vi "Newport ITX-D3N.vi"(5 "Disable Filter?":bool, 7 "Device Number (Display In Header)":string, 8 "error in (no error)":errorcluster, 10 "Remote Port":u16=2000, 11 "Machine":string="192.168.1.200") -> (0 "error out":errorcluster, 1 "iTHX/iBTHX Output":T1, 2 "Newport ITX Data":string[][](array[string]), 3 "Temp/Humidity":dbl[](array[numeric]))   [LabVIEW 2019]
doc: "Demonstrates how to display an interactive send and receive message dialog for communication between TCP connections. It establishes a connection on the machine listed and the port specified. It then waits for you to input data into the Input Line string control and hit enter. Once you hit enter, the string you typed is sent to the port and passed to the TCP Communicator - Passive.vi where it is displayed on a string indicator.\n\nThe key difference between the Active and Passive VIs is that the Active VI establishes a connection, while the Passive VI waits for a connection to be established.\n\n<B>Note:</B> Requires the TCP Communicator - Passive.vi."
uses:
  Type Definitions/iBTHX Data Values.ctl
panel:
  out "error out 2":errorcluster
  # "Instructions:\n1. Open the TCP\n    Communicator - Passive.vi\n    and run it first.\n2. Run TCP Communicator - \n    Active.vi second.\n3.Type into the Input Line\n    String Control and then\n    hit Enter.\n4. Type into the Input Line\n    of the other VI and then\n    hit Enter.\n5. Press Stop to end session."
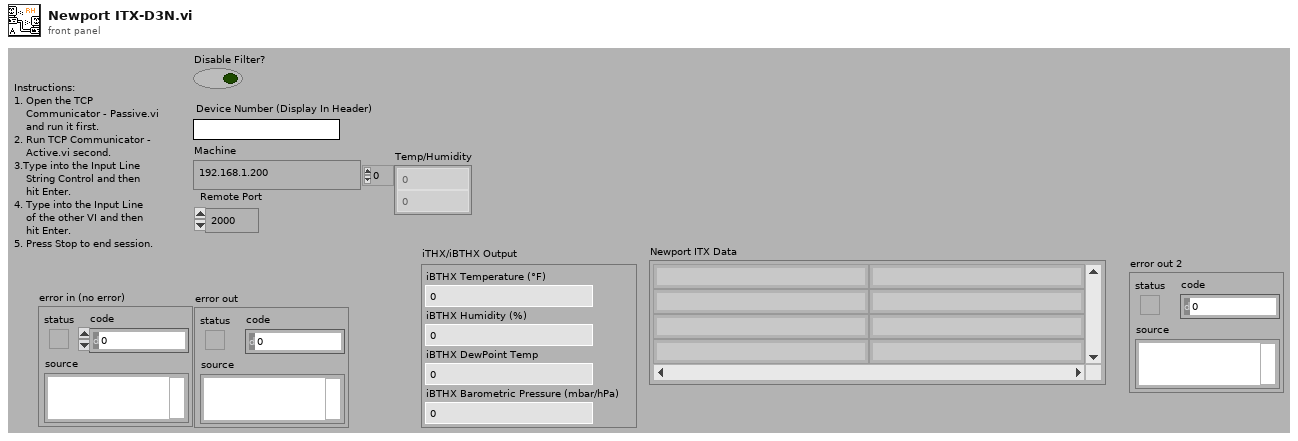
[diagram p1: front panel]
types:
  T1 = typedef "iBTHX Data Values.ctl" = cluster{"iBTHX Barometric Pressure (mbar/hPa)":dbl, "iBTHX Humidity (%)":dbl, "iBTHX Temperature (°F)":dbl, "iBTHX DewPoint Temp":dbl}
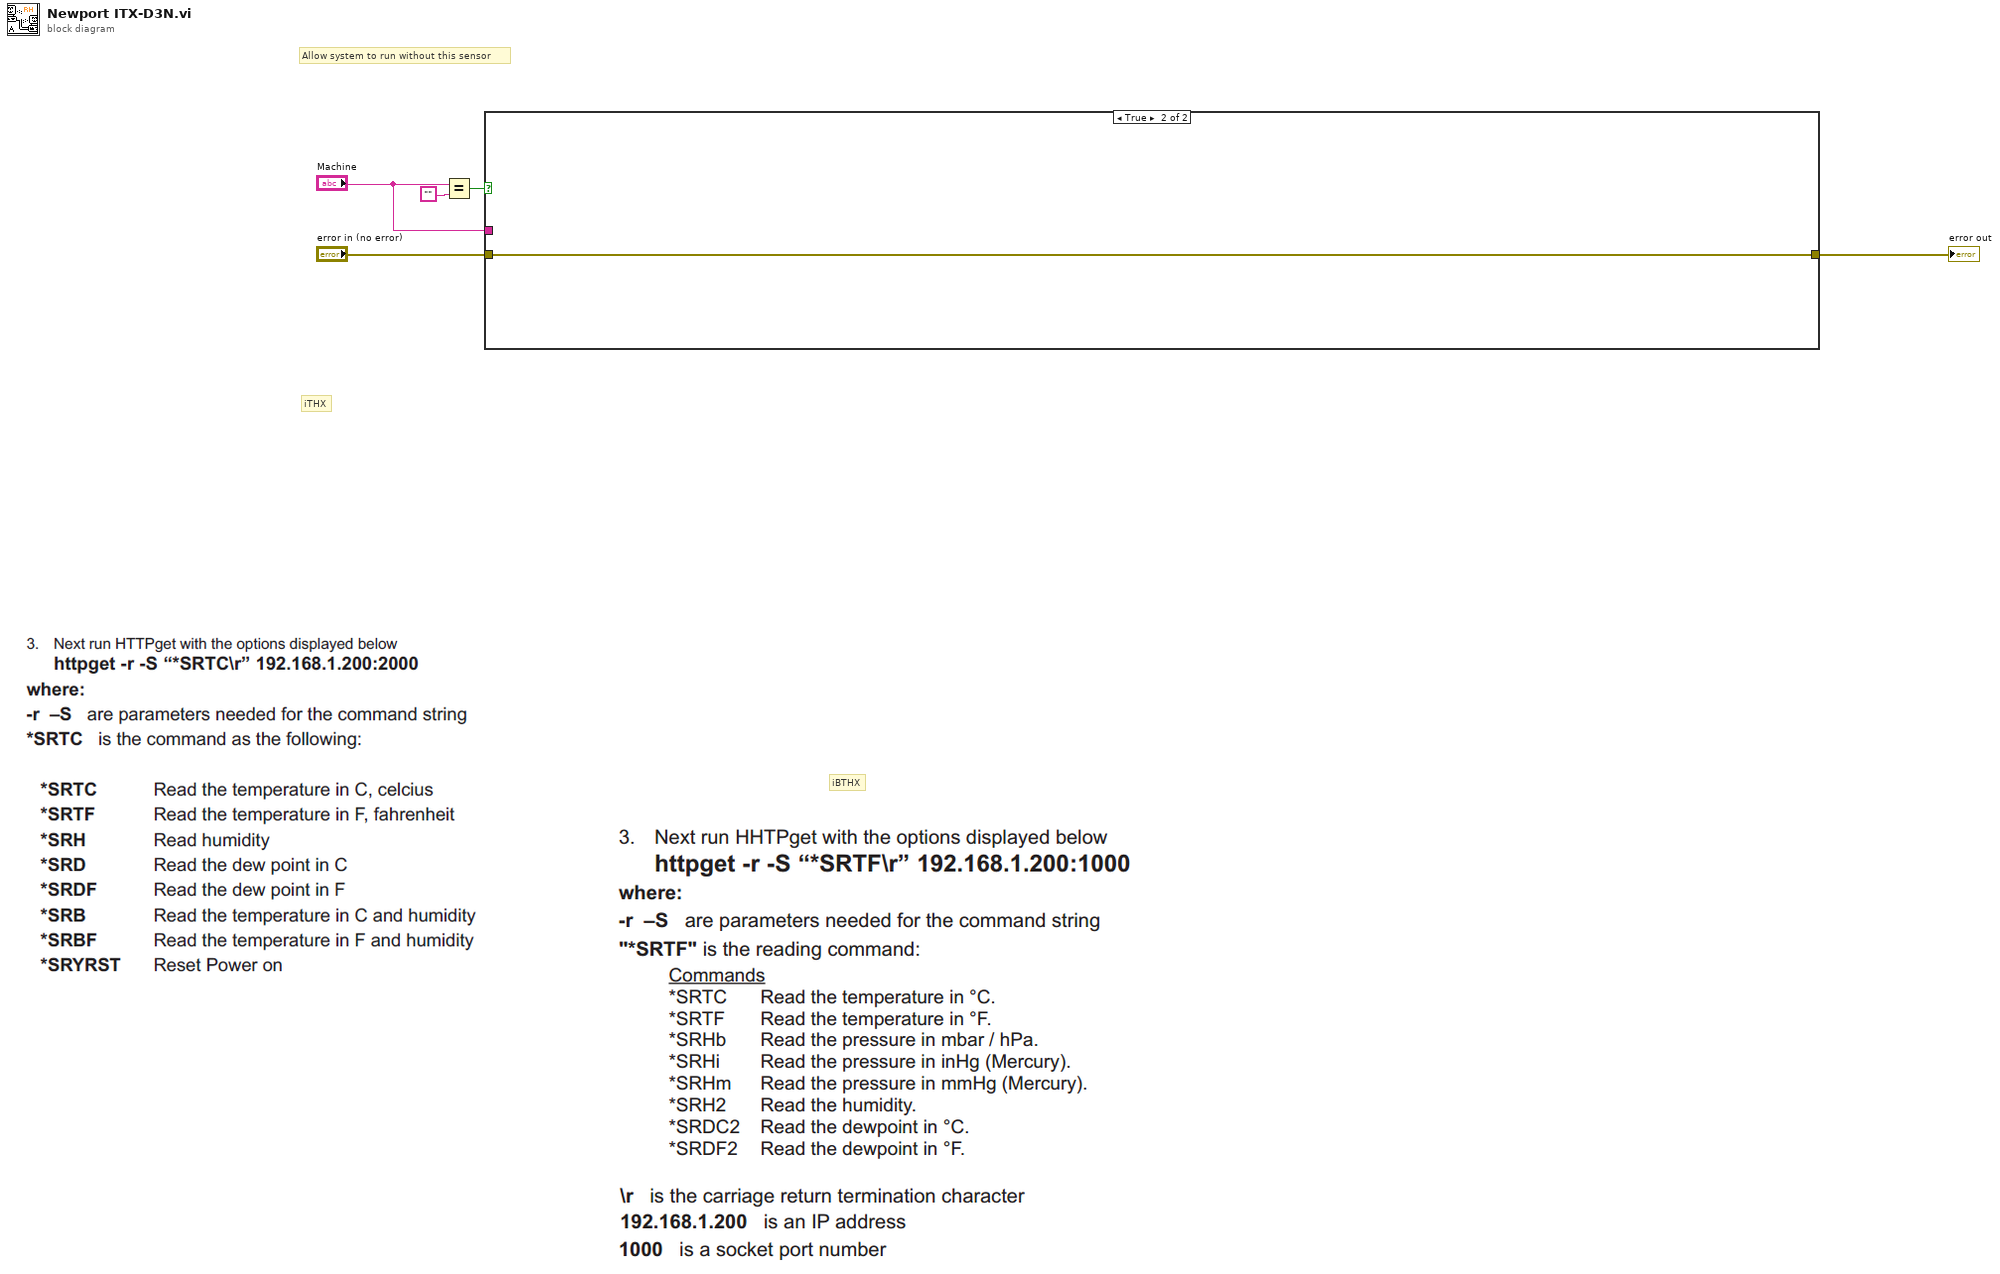
[diagram p0: block diagram]
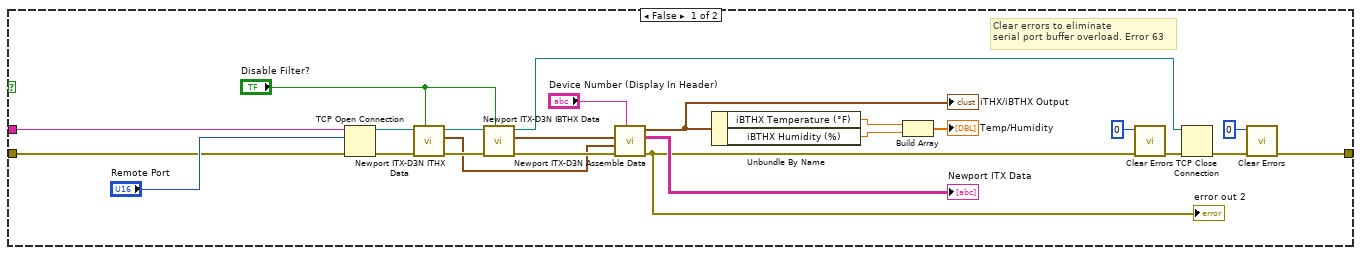
[diagram p2: hidden frame]
diagram:
  # "iTHX"
  # "iBTHX"
  # "Allow system to run without this sensor"
  n1 = Equal?(x="Machine", y="") -> (x = y?=w3:bool)
  n2 = case shown="True" w3 {
    tunnel: "Machine" -> [w29 _]
    tunnel: "error in (no error)" -> [w27 w30]
    tunnel: [w24 w30] -> w1
    frame False {
      # "Clear errors to eliminate\nserial port buffer overload. Error 63"
      n3 = TCP Open Connection(address=w29, remote port or service name="Remote Port", error in (no error)=w27) -> (connection ID=w20:refnum<k5>, error out=w21:errorcluster)  [unwired: 2 in]
      n4 = call "Newport ITX-D3N ITHX Data.vi"("Disable Filter?"="Disable Filter?", "error in (no error)"=w21, "TCP Network Connection in"=w20) -> ("error out"=w17:errorcluster, "ITHX Data"=w14:T1, "TCP Network Connection out"=w18:refnum<k5>)  [unwired: 6 in]
      n5 = call "Newport ITX-D3N IBTHX Data.vi"("Disable Filter?"="Disable Filter?", "error in (no error)"=w17, "TCP Network Connection in"=w18) -> ("error out"=w16:errorcluster, "iBTHX Data"=w15:T1, "TCP Network Connection out"=w19:refnum<k5>)  [unwired: 6 in]
      n6 = call "Newport ITX-D3N Assemble Data.vi"("Device Number (Display In Header)"="Device Number (Display In Header)", "Error In"=w16, "ITHX Data in"=w14, "iBTHX Data"=w15) -> ("Error Out"=w7:errorcluster, "Newport ITX Data"=→"Newport ITX Data":string[][], "ITHX Data out"=w13:T1)  [unwired: 5 in]
      "iTHX/iBTHX Output" <- w13
      "error out 2" <- w7
      n7 = Unbundle By Name(w13) -> ("iBTHX Temperature (°F)"=w12:dbl, "iBTHX Humidity (%)"=w11:dbl)
      n8 = Build Array(w12, w11) -> (→"Temp/Humidity":dbl[])
      n9 = call <vilib>:"Clear Errors.vi"("error in (no error)"=w7, "specific error code to clear (0: all)"=0) -> ("error out"=w22:errorcluster)  [unwired: 4 in, 1 out]
      n10 = TCP Close Connection(connection ID=w19, error in (no error)=w22) -> (error out=w25:errorcluster)  [unwired: 1 in, 1 out]
      n11 = call <vilib>:"Clear Errors.vi"("error in (no error)"=w25, "specific error code to clear (0: all)"=0) -> ("error out"=w24:errorcluster)  [unwired: 4 in, 1 out]
    }
    frame True {
    }
  }
  "error out" <- w1
